vi "Write Coordinates T+1.vi"(10 "Coordinates":T1, 11 "Movable in":refnum<class "Movable.lvclass">) -> (3 "Movable out":refnum<class "Movable.lvclass">)   [LabVIEW 2021, in "Movable.lvclass"]
doc: "MIT Licence\nCopyright (c) 2024 David Grollier"
uses:
  Movable.lvclass
  Type Def/Coordinates.ctl
  Movable.lvclass/Movable.ctl
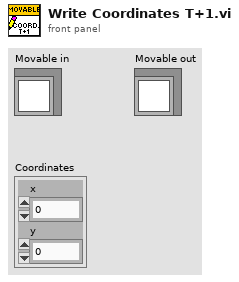
[diagram p1: front panel]
types:
  T1 = typedef "Coordinates.ctl" = cluster{"x":dbl, "y":dbl}
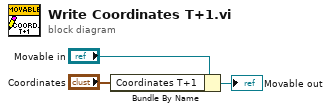
[diagram p0: block diagram]
diagram:
  n1 = Bundle By Name(cluster="Movable in", "Coordinates T+1"="Coordinates") -> (→"Movable out":refnum<class "Movable.lvclass">)
